vi "Arm Motor Movement.vi"(6 "Back Button":bool, 8 "RT":bool, 9 "LB":bool, 10 "RB":bool, 11 "Manuel Arm Motor Control":dbl format="%#_13g") -> ()   [LabVIEW 2020]
uses:
  <vilib>/Rock Robotics/WPI/ThirdParty/REV Robotics/REVLib/Typedef/Spark MAX Sensor Type.ctl
panel:
  in  "Arm Moter Set Value":dbl format="%#_13g"
  in  "Arm Motor Value":dbl format="%#_13g"
  out "Arrived At Setpoint":bool
  out "Arm Motor Position":dbl(graph)
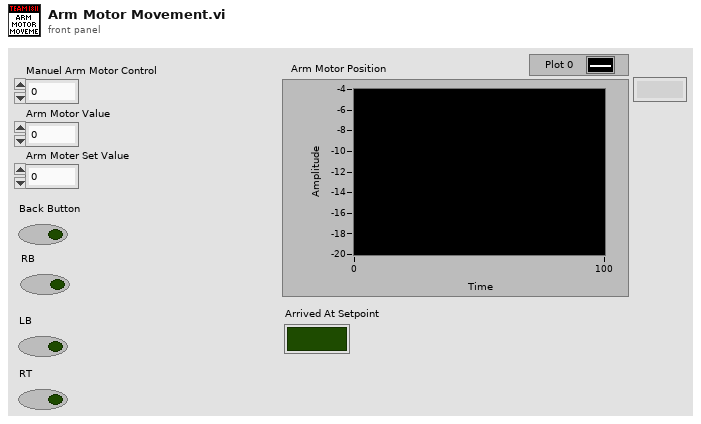
[diagram p1: front panel]
types:
  T1 = typedef "WPI_MotorControlDeviceRef.ctl" = cluster{"DeviceStatus":errorcluster, "Type":T2, "PWM":cluster{"PWM Channel":T3, "DeadBand":T4}, "CAN":cluster{"Device Number":u8, "SetOutput VI Ref":variant, "GetOutput VI Ref":variant, "Enable VI Ref":variant, "Disable VI Ref":variant, "Data":variant}, "Invert":bool, "DIO PWM":cluster{"PWM \"Enable\" Channel":T3, "DIOChannel":T5, "PWM Rate":dbl}}
  T2 = typedef "WPI_MotorControlType.ctl" = enum16{"PWM", "CAN", "DIO PWM"}
  T3 = typedef "FPGA_DIOPWMChannel.ctl" = enum8{"PWM 0", "PWM 1", "PWM 2", "PWM 3", "PWM 4", "PWM 5", "PWM 6", "PWM 7", "PWM 8", "PWM 9", "PWM MXP 0", "PWM MXP 1", "PWM MXP 2", "PWM MXP 3", "PWM MXP 4", "PWM MXP 5", "PWM MXP 6", "PWM MXP 7", "PWM MXP 8", "PWM MXP 9", "Invalid"}
  T4 = typedef "WPI_PWMDeadband.ctl" = cluster{"Name":string, "maxPositivePwm":i32, "minPositivePwm":i32, "centerPwm":i32, "maxNegativePwm":i32, "minNegativePwm":i32, "angularRange":u16}
  T5 = typedef "FPGA_DIOChannel.ctl" = enum8{"DIO 0", "DIO 1", "DIO 2", "DIO 3", "DIO 4", "DIO 5", "DIO 6", "DIO 7", "DIO 8", "DIO 9", "DIO MXP 0", "DIO MXP 1", "DIO MXP 2", "DIO MXP 3", "DIO MXP 4", "DIO MXP 5", "DIO MXP 6", "DIO MXP 7", "DIO MXP 8", "DIO MXP 9", "DIO MXP 10", "DIO MXP 11", "DIO MXP 12", "DIO MXP 13", "DIO MXP 14", "DIO MXP 15", "SPI Port CS1", "SPI Port CS2", "SPI Port CS3", "SPI Port MISO", "SPI Port MOSI", "Invalid"}
  T6 = typedef "Spark MAX Sensor Type.ctl" = enum16{"No Sensor", "Hall Sensor", "Encoder", "-Not Available-", "Analog", "Alternate Encoder", "Duty Cycle"}
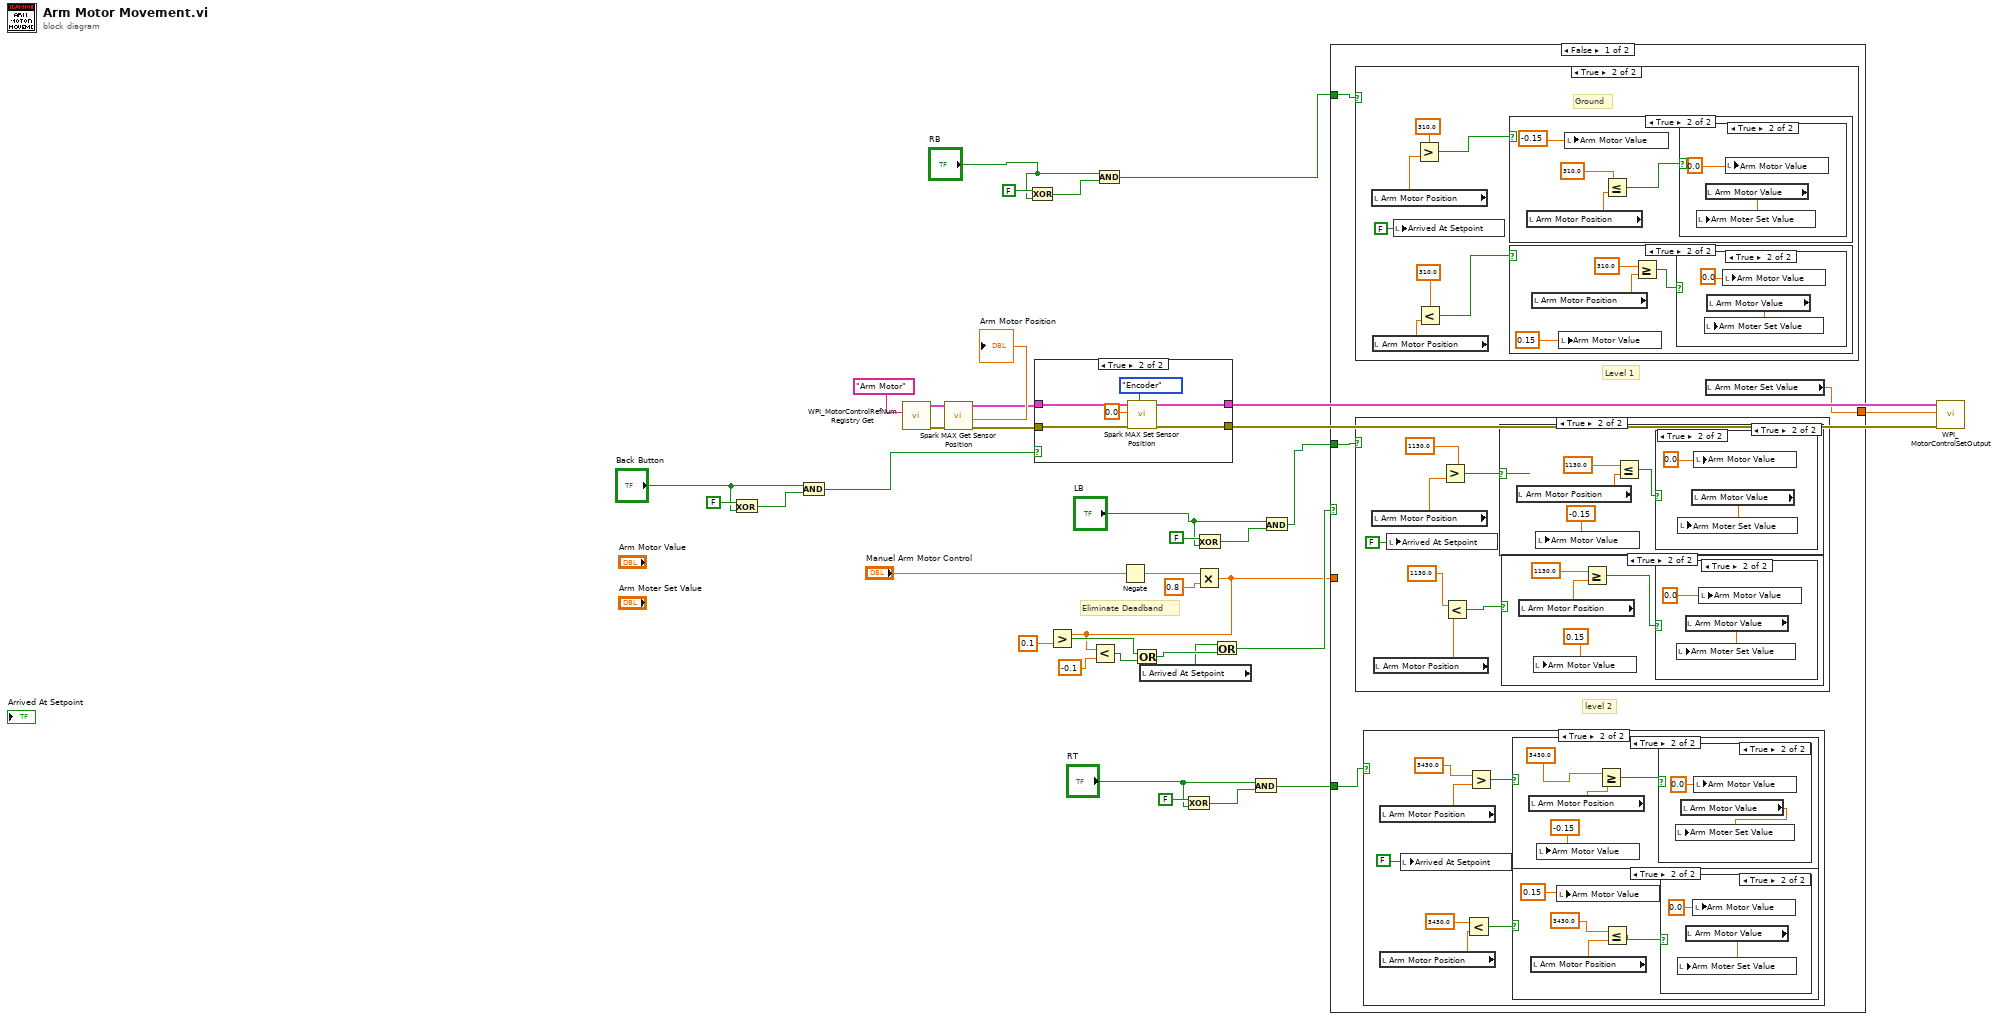
[diagram p0: block diagram]
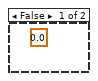
[diagram p12: hidden frame]
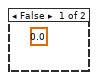
[diagram p15: hidden frame]
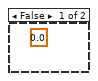
[diagram p16: hidden frame]
diagram:
  # "Eliminate Deadband"
  n1 = Exclusive Or(1:"Back Button", 2:FALSE ("x")) -> (0:w27:bool)
  n2 = And(x="Back Button", y=w27) -> (x .and. y?=w26:bool)
  n3 = call <vilib>:"WPI_MotorControlRefNum Registry Get.vi"("refnum name"="Arm Motor") -> ("error out"=w34:errorcluster, "MotorControlDevRef"=w35:T1)  [unwired: 9 in]
  n4 = call <vilib>:"Spark MAX Get Sensor Position.vi"("error in (no error)"=w34, "MotorControlDevRef in"=w35) -> ("error out"=w30:errorcluster, "Sensor Position"=→"Arm Motor Position":dbl, "MotorControlDevRef out"=w29:T1)  [unwired: 6 in, 1 out]
  n5 = Exclusive Or(1:"RB", 2:FALSE ("x")) -> (0:w9:bool)
  n6 = case shown="True" w26 {
    tunnel: [w37 w43] -> w31
    tunnel: w30 -> [w37 w44]
    tunnel: w29 -> [w38 w41]
    tunnel: [w38 w42] -> w32
    frame False {
    }
    frame True {
      n7 = call <vilib>:"Spark MAX Set Sensor Position.vi"("Sensor Type (Hall Sensor)"=Spark_MAX_Sensor_Type."Encoder", "error in"=w44, "Position"=0.0, "MotorControlDeviceRef"=w41) -> ("error out"=w43:errorcluster, "MotorControlDeviceRef"=w42:T1)  [unwired: 6 in]
    }
  }
  n8 = And(x="RB", y=w9) -> (x .and. y?=w3:bool)
  n9 = Negate(x="Manuel Arm Motor Control") -> (-x=w24:dbl)
  n10 = local read "Arrived At Setpoint"() -> (w17:bool)
  n11 = Exclusive Or(1:"RT", 2:FALSE ("x")) -> (0:w11:bool)
  n12 = Multiply(x=w24, y=0.8) -> (x*y=w13:dbl)
  n13 = Greater?(x=w13, y=0.1) -> (0:w20:bool)
  n14 = Less?(x=w13, y=-0.1) -> (x < y?=w21:bool)
  n15 = Or(x=w20, y=w21) -> (x .or. y?=w19:bool)
  n16 = Exclusive Or(1:"LB", 2:FALSE ("x")) -> (0:w7:bool)
  n17 = Or(x=w17, y=w19) -> (x .or. y?=w15:bool)
  n18 = And(x="RT", y=w11) -> (x .and. y?=w1:bool)
  n19 = And(x="LB", y=w7) -> (x .and. y?=w2:bool)
  n20 = case shown="False" w15 {
    tunnel: [w48 w106] -> w14
    tunnel: w13 -> [_ w106]
    tunnel: w3 -> [w47 _]
    tunnel: w2 -> [w46 _]
    tunnel: w1 -> [w45 _]
    frame False {
      # "Level 1"
      # "level 2"
      n21 = case shown="True" w47 {
        frame False {
          (unwired) 0.0
        }
        frame True {
          # "Ground"
          n22 = local read "Arm Motor Position"() -> (w90:dbl)
          n23 = local read "Arm Motor Position"() -> (w93:dbl)
          n24 = local write "Arrived At Setpoint"(FALSE) -> ()
          n25 = Greater?(x=310.0, y=w90) -> (0:w89:bool)
          n26 = Less?(x=310.0, y=w93) -> (x < y?=w88:bool)
          n27 = case shown="True" w89 {
            frame False {
              (unwired) 0.0
            }
            frame True {
              n28 = local read "Arm Motor Position"() -> (w102:dbl)
              n29 = local write "Arm Motor Value"(-0.15 ("Position Telloscoping arm")) -> ()
              n30 = Less Or Equal?(x=310.0, y=w102) -> (x <= y?=w100:bool)
              n31 = case shown="True" w100 {
                frame False {
                  (unwired) 0.0
                }
                frame True {
                  n32 = local read "Arm Motor Value"() -> (w104:dbl)
                  n33 = local write "Arm Moter Set Value"(w104) -> ()
                  n34 = local write "Arm Motor Value"(0.0 ("Arm Tellescope")) -> ()
                }
              }
            }
          }
          n35 = case shown="True" w88 {
            frame False {
            }
            frame True {
              n36 = local read "Arm Motor Position"() -> (w95:dbl)
              n37 = local write "Arm Motor Value"(0.15 ("Arm Movement")) -> ()
              n38 = Greater Or Equal?(x=310.0, y=w95) -> (x >= y?=w94:bool)
              n39 = case shown="True" w94 {
                frame False {
                }
                frame True {
                  n40 = local read "Arm Motor Value"() -> (w98:dbl)
                  n41 = local write "Arm Moter Set Value"(w98) -> ()
                  n42 = local write "Arm Motor Value"(0.0 ("Arm Tellescope")) -> ()
                }
              }
            }
          }
        }
      }
      n43 = case shown="True" w46 {
        frame False {
        }
        frame True {
          n44 = local read "Arm Motor Position"() -> (w70:dbl)
          n45 = local read "Arm Motor Position"() -> (w69:dbl)
          n46 = local write "Arrived At Setpoint"(FALSE) -> ()
          n47 = Greater?(x=1130.0, y=w70) -> (0:w71:bool)
          n48 = Less?(x=1130.0, y=w69) -> (x < y?=w72:bool)
          n49 = case shown="True" w71 {
            frame False {
            }
            frame True {
              n50 = local read "Arm Motor Position"() -> (w77:dbl)
              n51 = local write "Arm Motor Value"(-0.15) -> ()
              n52 = Less Or Equal?(x=1130.0, y=w77) -> (x <= y?=w75:bool)
              n53 = case shown="True" w75 {
                frame False {
                }
                frame True {
                  n54 = local read "Arm Motor Value"() -> (w79:dbl)
                  n55 = local write "Arm Moter Set Value"(w79) -> ()
                  n56 = local write "Arm Motor Value"(0.0) -> ()
                }
              }
            }
          }
          n57 = case shown="True" w72 {
            frame False {
            }
            frame True {
              n58 = local read "Arm Motor Position"() -> (w83:dbl)
              n59 = local write "Arm Motor Value"(0.15 ("Arm Motor Position")) -> ()
              n60 = Greater Or Equal?(x=1130.0, y=w83) -> (x >= y?=w81:bool)
              n61 = case shown="True" w81 {
                frame False {
                }
                frame True {
                  n62 = local read "Arm Motor Value"() -> (w85:dbl)
                  n63 = local write "Arm Moter Set Value"(w85) -> ()
                  n64 = local write "Arm Motor Value"(0.0 ("Position Telloscoping arm")) -> ()
                }
              }
            }
          }
        }
      }
      n65 = case shown="True" w45 {
        frame False {
        }
        frame True {
          n66 = local read "Arm Motor Position"() -> (w50:dbl)
          n67 = local read "Arm Motor Position"() -> (w52:dbl)
          n68 = local write "Arrived At Setpoint"(FALSE) -> ()
          n69 = Less?(x=3430.0, y=w52) -> (x < y?=w54:bool)
          n70 = Greater?(x=3430.0, y=w50) -> (0:w51:bool)
          n71 = case shown="True" w51 {
            frame False {
            }
            frame True {
              n72 = local read "Arm Motor Position"() -> (w59:dbl)
              n73 = local write "Arm Motor Value"(-0.15) -> ()
              n74 = Greater Or Equal?(x=3430.0, y=w59) -> (x >= y?=w56:bool)
              n75 = case shown="True" w56 {
                frame False {
                }
                frame True {
                  n76 = local read "Arm Motor Value"() -> (w60:dbl)
                  n77 = local write "Arm Moter Set Value"(w60) -> ()
                  n78 = local write "Arm Motor Value"(0.0) -> ()
                }
              }
            }
          }
          n79 = case shown="True" w54 {
            frame False {
            }
            frame True {
              n80 = local read "Arm Motor Position"() -> (w64:dbl)
              n81 = local write "Arm Motor Value"(0.15 ("Arm Motor Position")) -> ()
              n82 = Less Or Equal?(x=3430.0, y=w64) -> (x <= y?=w62:bool)
              n83 = case shown="True" w62 {
                frame False {
                }
                frame True {
                  n84 = local read "Arm Motor Value"() -> (w66:dbl)
                  n85 = local write "Arm Moter Set Value"(w66) -> ()
                  n86 = local write "Arm Motor Value"(0.0 ("Position Telloscoping arm")) -> ()
                }
              }
            }
          }
        }
      }
      n87 = local read "Arm Moter Set Value"() -> (w48:dbl)
    }
    frame True {
      # "Give Control To Driver Joystick"
    }
  }
  n88 = call <vilib>:"WPI_MotorControlSetOutput.vi"("error in (no error)"=w31, "Output"=w14, "MotorControlDevRef"=w32) -> ()  [unwired: 6 in, 3 out]
